vi "test_U8 Write and Read.vi"(8 "error in (no error)":errorcluster, 11 "Scalar Channels Testing in":refnum<class "FPGA Addon Scalar Channels System Tests.lvclass">=refnum) -> (0 "error out":errorcluster, 3 "Scalar Channels Testing out":refnum<class "FPGA Addon Scalar Channels System Tests.lvclass">)   [LabVIEW 2019, in "FPGA Addon Scalar Channels System Tests.lvclass"]
uses:
  FPGA Addon Scalar Channels System Tests.lvclass
  FPGA Addon Test Class/FPGA Addon Test Class.lvclass
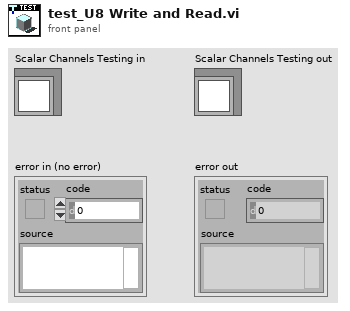
[diagram p1: front panel]
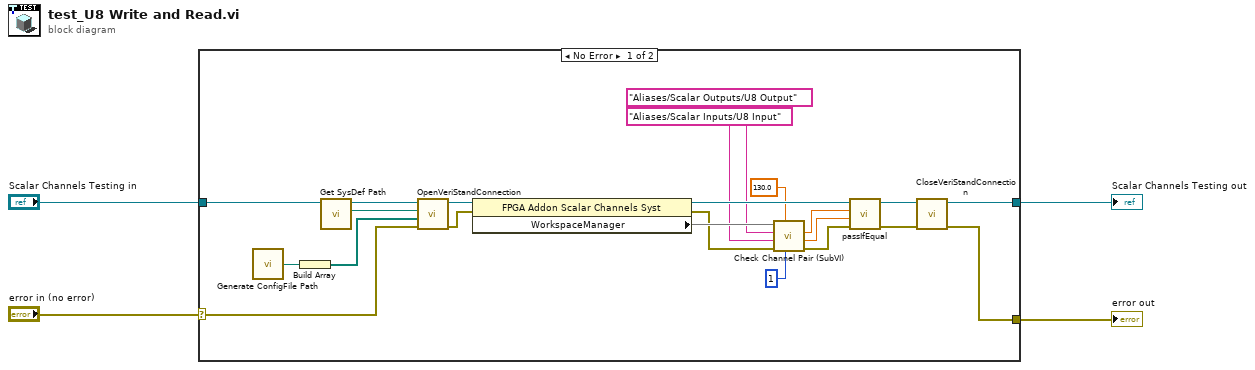
[diagram p0: block diagram]
diagram:
  n1 = case shown="No Error" "error in (no error)" {
    selector: "error in (no error)" -> [w19 w28]
    tunnel: [w25 w28] -> w3
    tunnel: [w26 w27] -> w1
    tunnel: "Scalar Channels Testing in" -> [w18 w27]
    frame No Error {
      n2 = call "Generate ConfigFile Path.vi"() -> ("ConfigFile path"=w7:path)
      n3 = Build Array(w7) -> (w6:path[])
      n4 = call "Get SysDef Path.vi"("Scalar Channels Testing in"=w18) -> ("SysDef Path"=w16:path, "Scalar Channels Testing out"=w17:refnum<class "FPGA Addon Test Class.lvclass">)  [unwired: 9 in]
      n5 = call-dynamic "OpenVeriStandConnection.vi"("error in (no error)"=w19, "overrides files"=w6, "System Definition File"=w16, "VeriStand Test Case in"=w17) -> ("error out"=w24:errorcluster, "VeriStand Test Case out"=w23:refnum<class "FPGA Addon Scalar Channels System Tests.lvclass">)  [unwired: 5 in, 1 out]
      n6 = property class="FPGA Addon Scalar Channels Syst"(reference=w23, error in=w24) -> (reference out=w22:refnum<class "FPGA Addon Scalar Channels System Tests.lvclass">, error out=w12:errorcluster, "WorkspaceManager"=w15)
      n7 = call "Check Channel Pair (SubVI).vi"("seconds to wait"=u32 1 ("milliseconds to wait"), "OutputChannel Value in"=130.0 ("Value"), "error in (no error)"=w12, "Input Channel"="Aliases/Scalar Inputs/U8 Input" ("Channel"), "Output Channel"="Aliases/Scalar Outputs/U8 Output" ("Channel"), "WorkspaceManager in"=w15) -> ("error out"=w13:errorcluster, "OutputChannel Value out"=w8:dbl, "InputChanel Value"=w9:dbl)  [unwired: 2 in, 1 out]
      n8 = call-dynamic "passIfEqual.vi"("error in (no error)"=w13, "y"=w8, "x"=w9, "TestCase in"=w22) -> ("error out"=w20:errorcluster, "TestCase out"=w21:refnum<class "FPGA Addon Scalar Channels System Tests.lvclass">)  [unwired: 6 in]
      n9 = call-dynamic "CloseVeriStandConnection.vi"("error in (no error)"=w20, "VeriStand Test Case in"=w21) -> ("error out"=w25:errorcluster, "VeriStand Test Case out"=w26:refnum<class "FPGA Addon Scalar Channels System Tests.lvclass">)  [unwired: 8 in]
    }
    frame Error {
    }
  }
  "error out" <- w3
  "Scalar Channels Testing out" <- w1
